vi "knob.vi"() -> ()   [LabVIEW 2021]
panel:
  in  "Knob":dbl(knob) scale=0.0..100.0
  in  "stop":bool
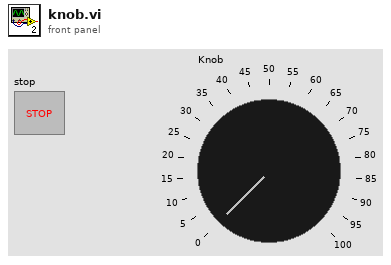
[diagram p1: front panel]
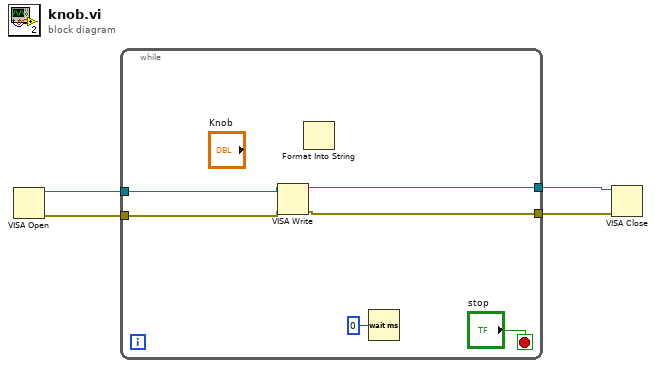
[diagram p0: block diagram]
diagram:
  n1 = VISA Open() -> (VISA resource name=w4:refnum<visa-resource-name>, error out=w3:errorcluster)  [unwired: 5 in]
  n2 = while {
    tunnel: w4 -> [w8]
    tunnel: w3 -> [w7]
    tunnel: [w6] -> w2
    tunnel: [w5] -> w1
    stop <- "stop" stop-if-true
    n3 = VISA Write(VISA resource name=w8, error in (no error)=w7) -> (VISA resource name out=w6:refnum<visa-resource-name>, error out=w5:errorcluster)  [unwired: 1 in, 1 out]
    n4 = Format Into String() -> ()  [unwired: 4 in, 2 out]
    n5 = Wait (ms)(milliseconds to wait=u32 0) -> ()  [unwired: 1 out]
  }
  n6 = VISA Close(VISA resource name=w2, error in (no error)=w1) -> ()  [unwired: 1 out]
